vi "Destroy.vi"(8 "error in (no error)":errorcluster, 11 "RTFIFODouble in":refnum<class "CIFTag.lvclass">) -> (0 "error out":errorcluster, 3 "RTFIFODouble out":refnum<class "CIFTag.lvclass">)   [LabVIEW 2021, in "CIFTag.lvclass"]
uses:
  CIFTag.lvclass
  CIFTag.lvclass/CIFTag.ctl
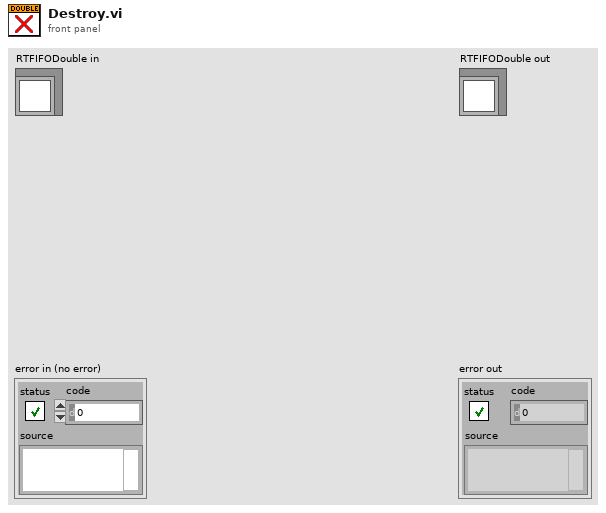
[diagram p1: front panel]
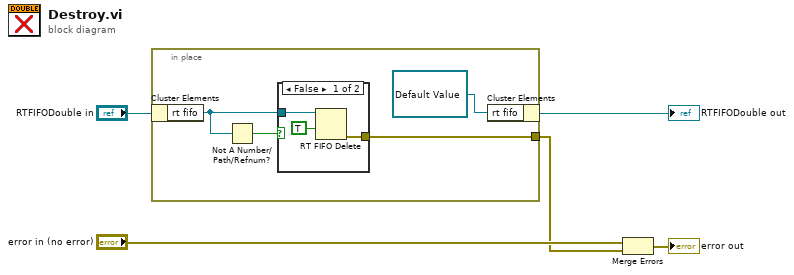
[diagram p0: block diagram]
diagram:
  n1 = in-place {
    in-place-border: [w6] -> w2
    n2 = in-place-cluster #1("RTFIFODouble in") -> ("rt fifo"=w8:refnum<k33>)
    n3 = Not A Number/Path/Refnum?(number/path/refnum=w8) -> (NaN/Path/Refnum?=w9:bool)
    n4 = case shown="False" w9 {
      tunnel: w8 -> [w12 _]
      tunnel: [w11 _] -> w6
      frame False {
        n5 = RT FIFO Delete(0:w12, 2:TRUE ("force destroy? (F)")) -> (11:w11:errorcluster)  [unwired: 1 in]
      }
      frame True {
      }
    }
    n6 = in-place-cluster #1("rt fifo"=refnum<k33> refnum) -> (→"RTFIFODouble out":refnum<class "CIFTag.lvclass">)
  }
  n7 = Merge Errors("error in (no error)", w2) -> (→"error out":errorcluster)
